vi "Write Y.vi"(8 "error in (no error)":errorcluster, 10 "Y":i32, 11 "Cautious Wolf in":refnum<class "Cautious Wolf.lvclass">) -> (0 "error out":errorcluster, 3 "Cautious Wolf out":refnum<class "Cautious Wolf.lvclass">)   [LabVIEW 2020, in "Cautious Wolf.lvclass"]
uses:
  Cautious Wolf.lvclass
  Cautious Wolf.lvclass/Cautious Wolf.ctl
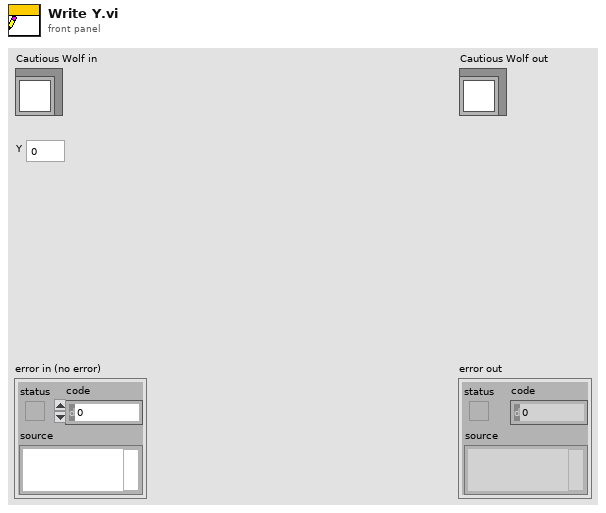
[diagram p1: front panel]
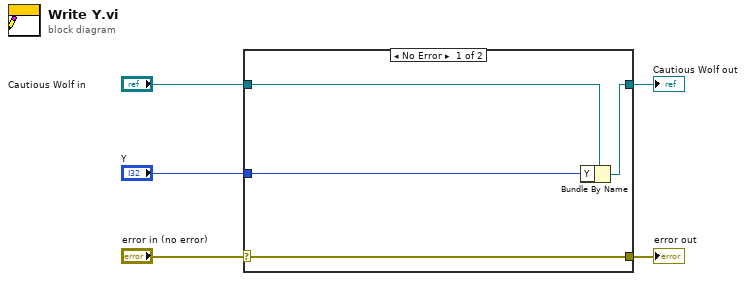
[diagram p0: block diagram]
diagram:
  n1 = case shown="No Error" "error in (no error)" {
    selector: "error in (no error)" -> [w9 w10]
    tunnel: [w9 w10] -> w4
    tunnel: [w7 w11] -> w2
    tunnel: "Cautious Wolf in" -> [w8 w11]
    tunnel: "Y" -> [w6 _]
    frame No Error {
      n2 = Bundle By Name(cluster=w8, "Y"=w6) -> (w7:refnum<class "Cautious Wolf.lvclass">)
    }
    frame Error {
    }
  }
  "error out" <- w4
  "Cautious Wolf out" <- w2
